vi "Convert Acceleration Units to Device Units.vi"(9 "Microstep Size (0)":dbl, 10 "Units (0: device acceleration units)":u16(ring) items=["device acceleration units", "microsteps per second squared", "microns per second squared", "millimeters per second squared", "inches per second squared", "degrees per second squared"], 11 "Acceleration (0)":dbl) -> (1 "Device Acceleration (64-bit)":i64, 2 "Device Acceleration (String)":string, 3 "Device Acceleration (32-bit)":i32)   [LabVIEW 2015, in "Zaber A Series.lvlib"]
doc: "Helper to convert standard units of acceleration to device-specific acceleration units.\n\nSelect a unit to convert from and enter an Acceleration quantity. \n\nIf you select a unit other than device units or microsteps per second squared, you must also provide the Microstep Size conversion factor from microsteps to micrometers (for linear devices) or degrees (for rotary devices), which can be found in your device manual.\n\nThis VI is deprecated in order to make the unit list consistent with the speed and position conversion VIs. Please use \"Convert Acceleration to Device Units' instead."
uses:
  Zaber A Series.lvlib
panel:
  # "DEPRECATED\n \n This VI is deprecated in order to make the unit list consistent with\n other VIs.  Please use the new \"Convert Acceleration to Device\n Units\" VI instead."
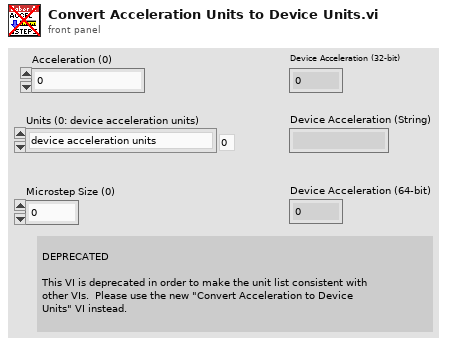
[diagram p1: front panel]
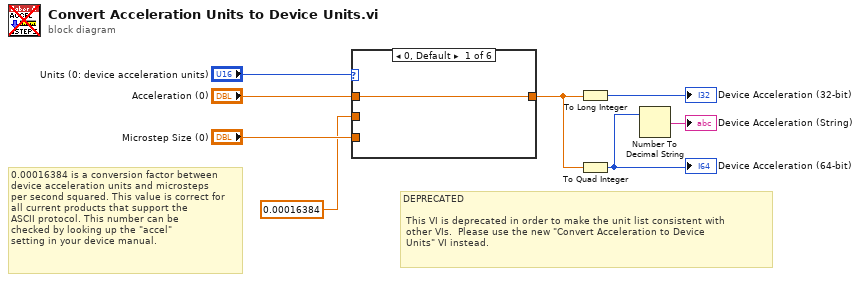
[diagram p0: block diagram]
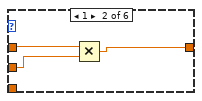
[diagram p2: hidden frame]
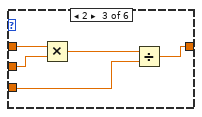
[diagram p3: hidden frame]
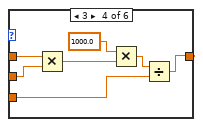
[diagram p4: hidden frame]
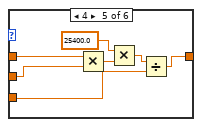
[diagram p5: hidden frame]
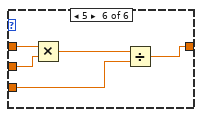
[diagram p6: hidden frame]
diagram:
  # "DEPRECATED\n \n This VI is deprecated in order to make the unit list consistent with\n other VIs.  Please use the new \"Convert Acceleration to Device\n Units\" VI instead."
  # "0.00016384 is a conversion factor between \ndevice acceleration units and microsteps \nper second squared. This value is correct for\nall current products that support the\nASCII protocol. This number can be \nchecked by looking up the \"accel\"\nsetting in your device manual."
  n1 = case shown="0, Default" "Units (0: device acceleration units)" {
    tunnel: 0.00016384 ("Acceleration Constant (0.00016384)") -> [_ w11 w16 w21 w30 w33]
    tunnel: "Microstep Size (0)" -> [_ _ w15 w20 w29 w32]
    tunnel: "Acceleration (0)" -> [w9 w12 w17 w22 w31 w34]
    tunnel: [w9 w10 w14 w18 w28 w35] -> w1
    frame 0, Default {
    }
    frame 1 {
      n2 = Multiply(x=w12, y=w11) -> (x*y=w10:dbl)
    }
    frame 2 {
      n3 = Multiply(x=w17, y=w16) -> (x*y=w13:dbl)
      n4 = Divide(x=w13, y=w15) -> (x/y=w14:dbl)
    }
    frame 3 {
      n5 = Multiply(x=w22, y=w21) -> (x*y=w19:dbl)
      n6 = Multiply(x=1000.0, y=w19) -> (x*y=w24:dbl)
      n7 = Divide(x=w24, y=w20) -> (x/y=w18:dbl)
    }
    frame 4 {
      n8 = Multiply(x=w31, y=w30) -> (x*y=w26:dbl)
      n9 = Multiply(x=25400.0, y=w26) -> (x*y=w25:dbl)
      n10 = Divide(x=w25, y=w29) -> (x/y=w28:dbl)
    }
    frame 5 {
      n11 = Multiply(x=w34, y=w33) -> (x*y=w36:dbl)
      n12 = Divide(x=w36, y=w32) -> (x/y=w35:dbl)
    }
  }
  n13 = To Long Integer(number=w1) -> (32bit integer=→"Device Acceleration (32-bit)":i32)
  n14 = To Quad Integer(1:w1) -> (0:w2:i64)
  "Device Acceleration (64-bit)" <- w2
  n15 = Number To Decimal String(number=w2) -> (decimal integer string=→"Device Acceleration (String)":string)  [unwired: 1 in]
